vi "웹서버 불리언값 출력.vi"(9 "lines":tag caption="라인", 11 "client handle":T1 caption="클라이언트 핸들") -> (0 "headers 4":string caption="연결확인 메세지 출력", 1 "y 3":u32, 2 "10진수 문자열":string[](array[string]), 3 "참조 번호 출력":T1 caption="client handle out", 5 "data":bool[](array[boolean]) caption="데이터", 6 "불리언값":string)   [LabVIEW 2019]
uses:
  <vilib>/httpClient/ClientHandle.ctl
  <vilib>/DAQmx/read.llb/DAQmx Read (Digital 1D Bool NChan 1Samp 1Line).vi
  <vilib>/DAQmx/create/channels.llb/DAQmx Create Channel (DI-Digital Input).vi
  <vilib>/DAQmx/configure/timing.llb/DAQmx Timing (Sample Clock).vi
  <vilib>/DAQmx/miscellaneous.llb/DAQmx Fill In Error Info.vi
  <vilib>/httpClient/PUTBuffer.vi
  <vilib>/httpClient/LabVIEWHTTPClient.lvlib
panel:
  out "error out":errorcluster
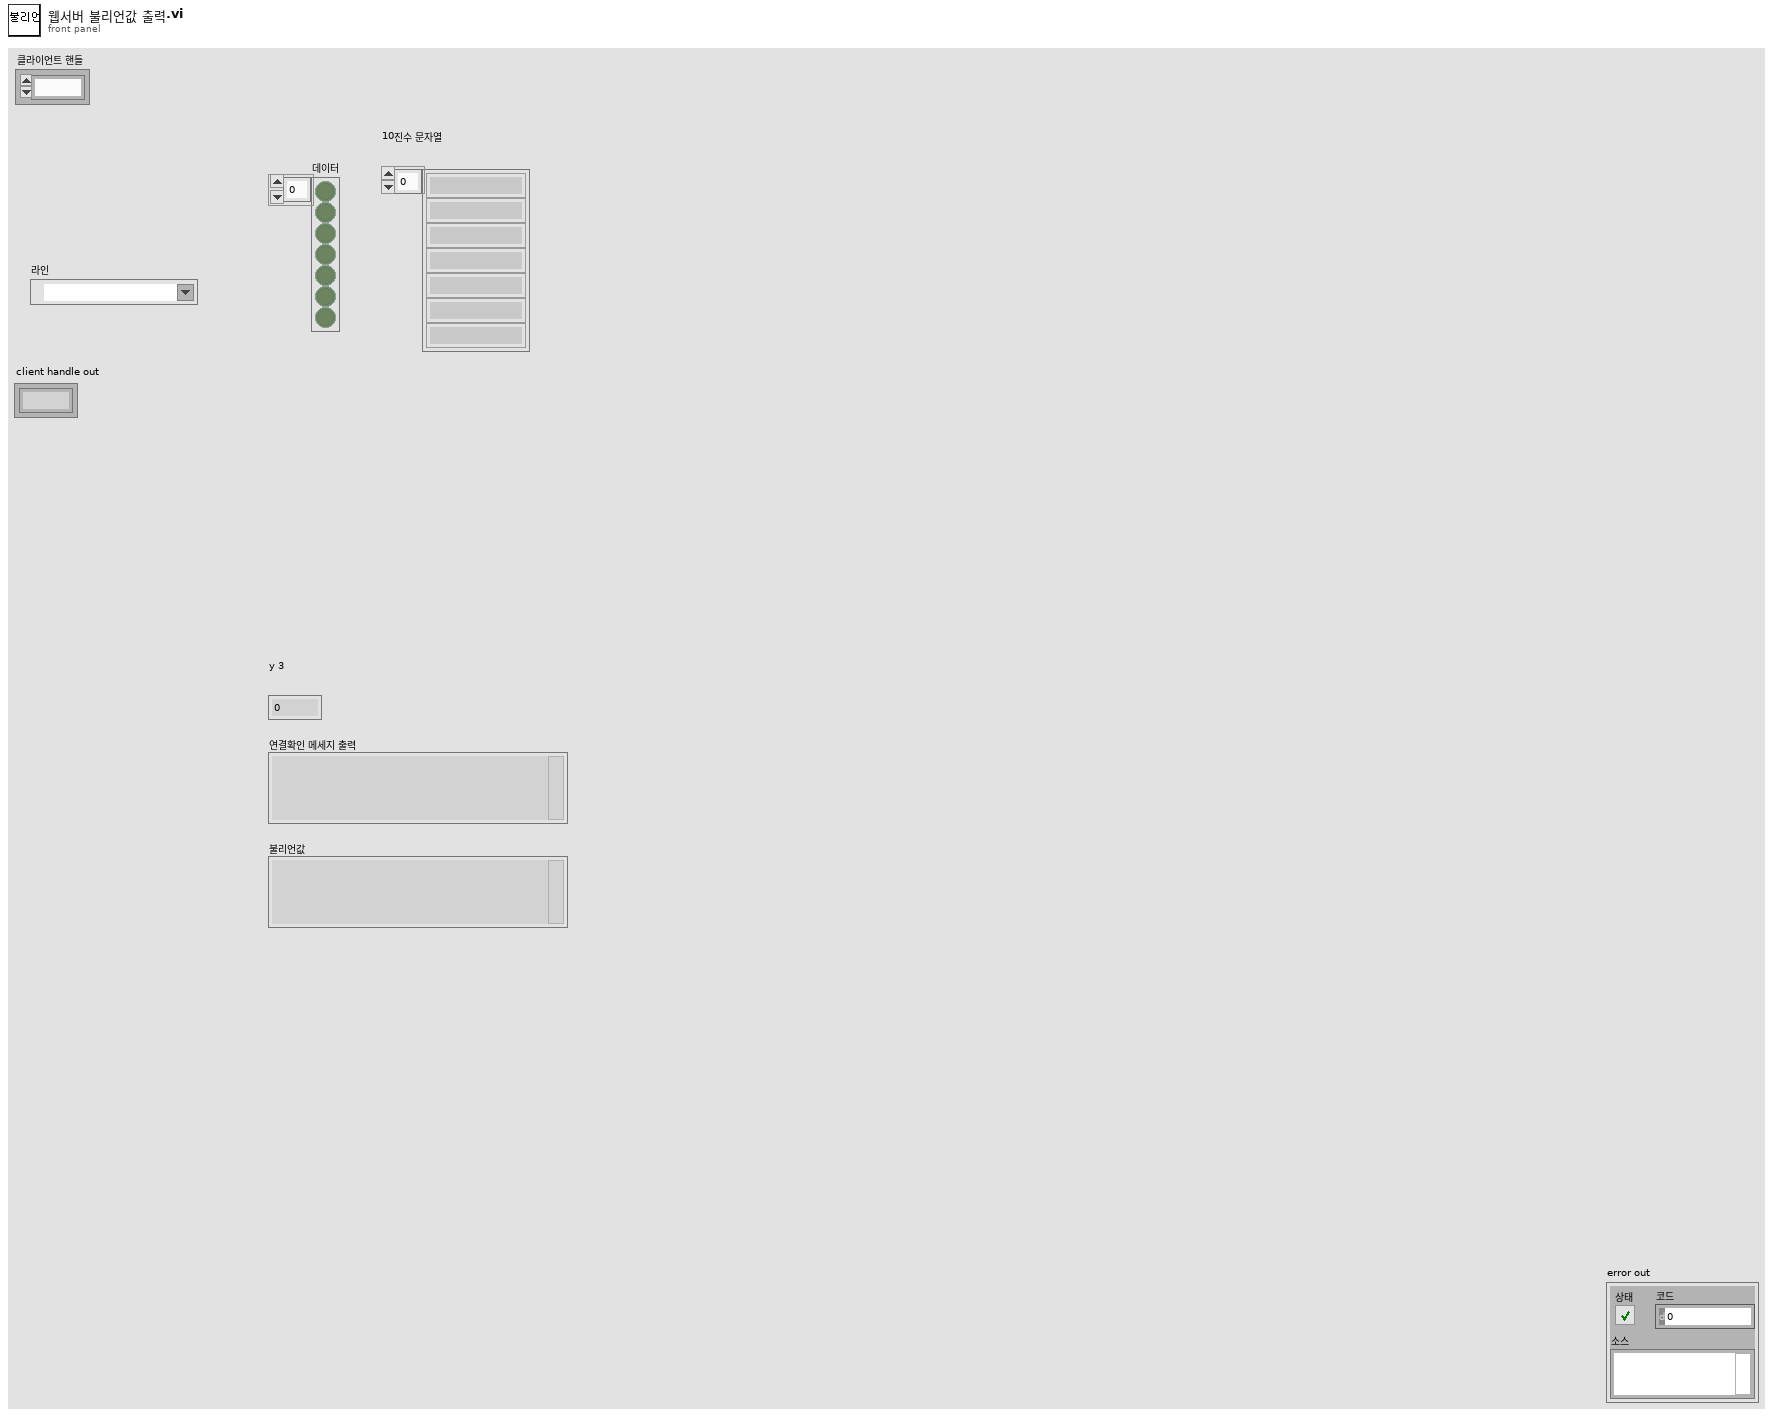
[diagram p1: front panel]
types:
  T1 = typedef "LabVIEWHTTPClient.lvlib/ClientHandle.ctl" = refnum<k1>
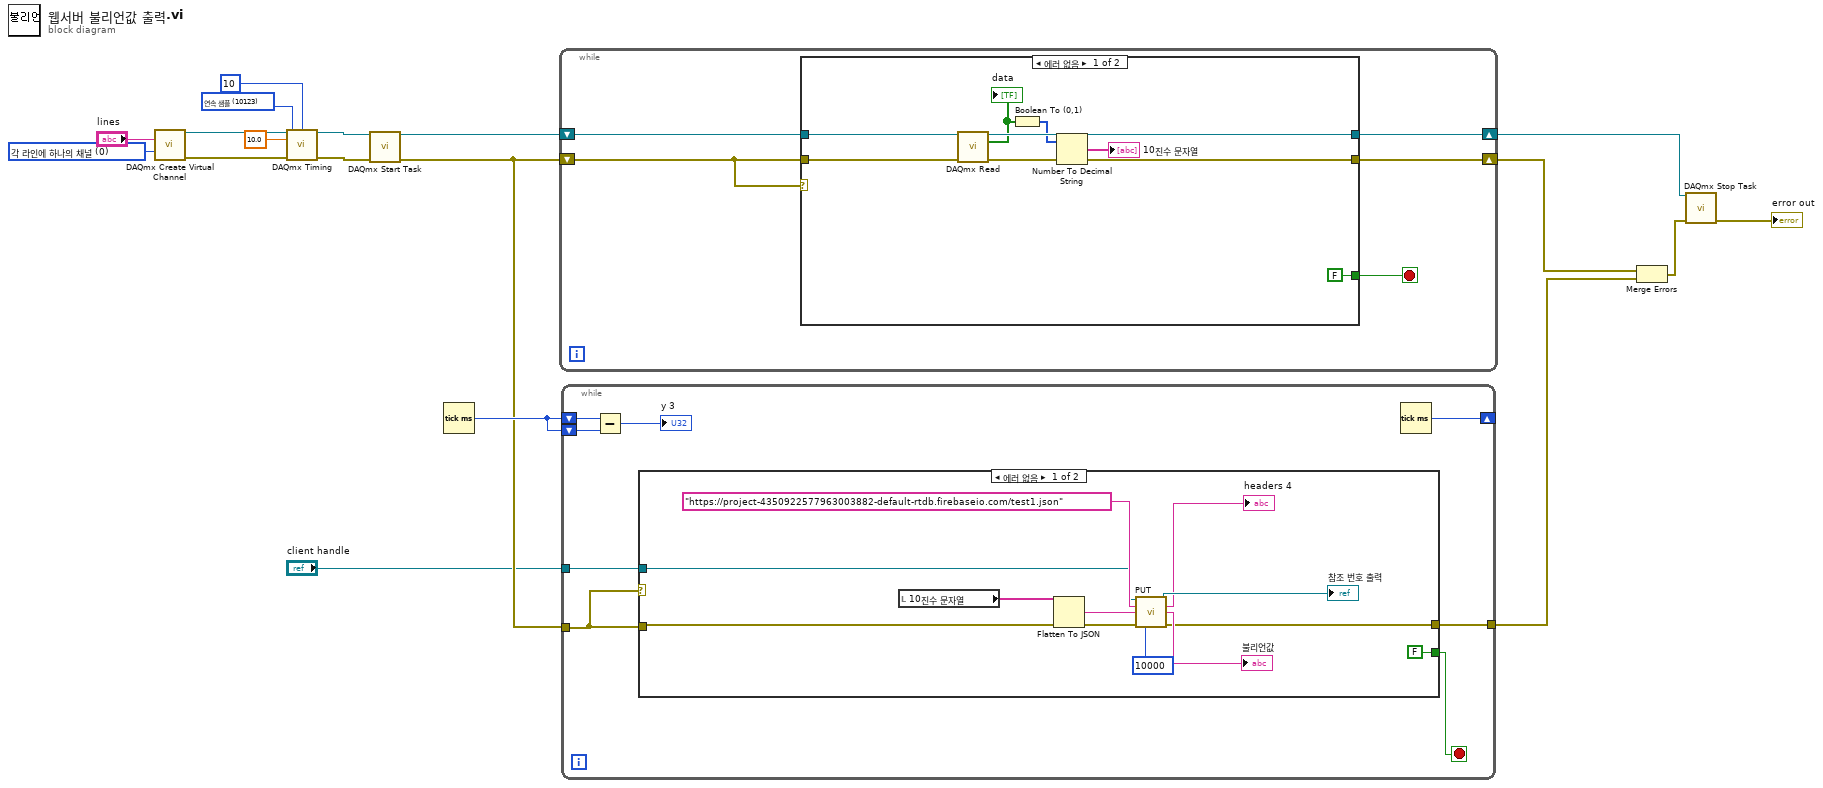
[diagram p0: block diagram]
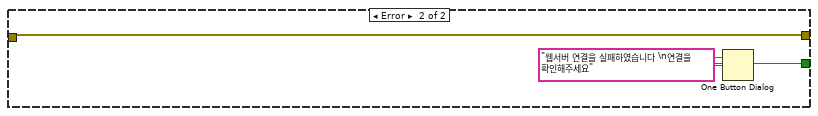
[diagram p2: hidden frame]
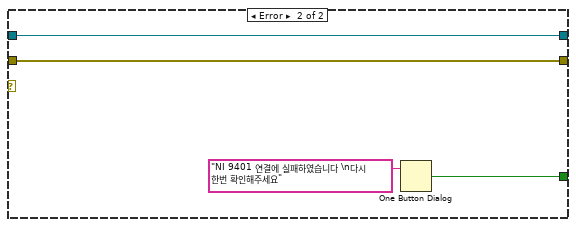
[diagram p3: hidden frame]
diagram:
  w9 = 10123 items=["유한 샘플"=10178, "연속 샘플"=10123, "하드웨어 타이밍에 의한 단일 포인트"=12522] ("sample mode")
  w8 = 0 items=["각 라인에 하나의 채널", "모든 라인에 하나의 채널"] ("line grouping")
  n1 = call-poly <vilib>:"DAQmx Create Virtual Channel.vi"("lines"="lines", "line grouping"=w8) -> ("task out"=w18:refnum<k21>, "error out"=w11:errorcluster)  [unwired: 12 in]
  n2 = call-poly <vilib>:"DAQmx Timing.vi"("task/channels in"=w18, "sample mode"=w9, "samples per channel"=10, "rate"=10.0, "error in"=w11) -> ("task out"=w12:refnum<k21>, "error out"=w13:errorcluster)  [unwired: 9 in]
  n3 = call <vilib>:"DAQmx Start Task.vi"("task/channels in"=w12, "error in"=w13) -> ("task out"=w7:refnum<k21>, "error out"=w14:errorcluster)  [unwired: 12 in]
  n4 = Tick Count (ms)() -> (millisecond timer value=w17:u32)
  n5 = while {
    shift-right: [w22] -> w1
    shift-left: w7 -> [w23]
    shift-right: [w21] -> w3
    shift-left: w14 -> [w20]
    stop <- w19 stop-if-true
    n6 = case shown="에러 없음" w20 {
      tunnel: w23 -> [w31 w34]
      tunnel: w20 -> [w30 w33]
      tunnel: [w29 w34] -> w22
      tunnel: [w28 w33] -> w21
      tunnel: [FALSE ("true") w32] -> w19
      frame No Error {
        n7 = call-poly <vilib>:"DAQmx Read.vi"("task/channels in"=w31, "error in"=w30) -> ("task out"=w29:refnum<k21>, "data"=w26:bool[], "error out"=w28:errorcluster)  [unwired: 11 in]
        "data" <- w26
        n8 = Boolean To (0,1)(Boolean=w26) -> (0, 1=w25:i16[])
        n9 = Number To Decimal String(number=w25) -> (decimal integer string=→"10진수 문자열":string[])  [unwired: 1 in]
      }
      frame Error {
        n10 = One Button Dialog(message="NI 9401 연결에 실패하였습니다 \n다시 한번 확인해주세요" ("메시지")) -> (true=w32:bool)  [unwired: 1 in]
      }
    }
  }
  n11 = while {
    tunnel: [w43] -> w2
    tunnel: w14 -> [w42]
    shift-right: [w40] -> _
    shift-left: w17 -> [w38]
    shift-left: w17 -> [w37]
    tunnel: "client handle" -> [w36]
    stop <- w41 stop-if-true
    n12 = Subtract(x=w38, y=w37) -> (x-y=→"y 3":u32)
    n13 = case shown="에러 없음" w42 {
      tunnel: w42 -> [w48 w57]
      tunnel: [w47 w57] -> w43
      tunnel: [FALSE ("true") w56] -> w41
      tunnel: w36 -> [w44 _]
      frame No Error {
        n14 = local read "10진수 문자열"() -> (w45:string[])
        n15 = Flatten To JSON(anything=w45, error in (no error)=w48) -> (JSON string=w52:string, 11:w51:errorcluster)  [unwired: 1 in]
        n16 = call-poly <vilib>:"PUT.vi"("client handle"=w44, "url"="https://project-4350922577963003882-default-rtdb.firebaseio.com/test1.json", "buffer"=w52, "error in (no error)"=w51, "timeout (10000)"=10000) -> ("client handle out"=→"참조 번호 출력":T1, "headers"=→"headers 4":string, "body"=→"불리언값":string, "error out"=w47:errorcluster)  [unwired: 7 in]
      }
      frame Error {
        n17 = One Button Dialog(message="웹서버 연결을 실패하였습니다 \n연결을 확인해주세요" ("메시지")) -> (true=w56:bool)  [unwired: 1 in]
      }
    }
    n18 = Tick Count (ms)() -> (millisecond timer value=w40:u32)
  }
  n19 = Merge Errors(w3, w2) -> (w4:errorcluster)
  n20 = call <vilib>:"DAQmx Stop Task.vi"("task/channels in"=w1, "error in"=w4) -> ("error out"=→"error out":errorcluster)  [unwired: 12 in, 1 out]
